vi "SQLite Get Table Names.vi"(8 "error in":errorcluster, 11 "SQLite Connection":refnum<class "Connection.lvclass">) -> (0 "error out":errorcluster, 2 "Table Names":string[](array[string]), 3 "Dup SQLite Connection":refnum<class "Connection.lvclass">)   [LabVIEW 2021, in "EDT SQLite+.lvlib"]
uses:
  EDT SQLite+.lvlib
  <vilib>/drjdpowell/SQLite Library/SQL Connection/Connection.lvclass
  <vilib>/drjdpowell/SQLite Library/SQL Statement/SQL Statement.lvclass/SQL Statement.ctl
  <vilib>/drjdpowell/SQLite Library/SQL Statement/Error Message.vi
  <vilib>/drjdpowell/SQLite Library/SQL Statement/Column String.vi
  <vilib>/drjdpowell/SQLite Library/SQL Statement/SQL Statement.lvclass
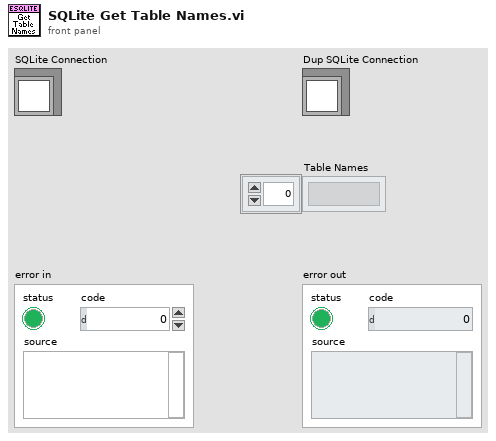
[diagram p1: front panel]
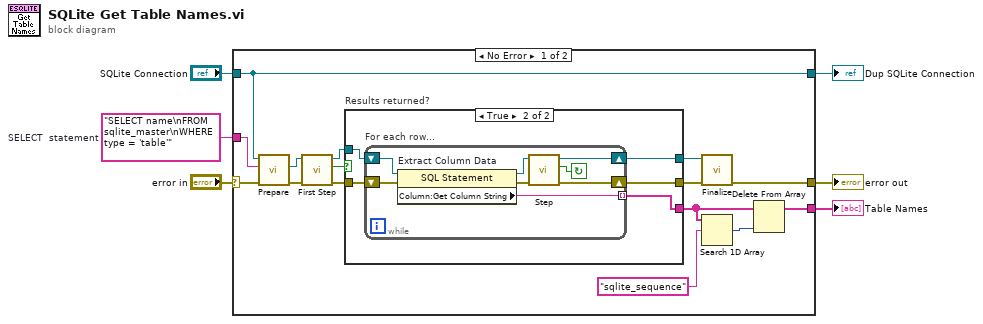
[diagram p0: block diagram]
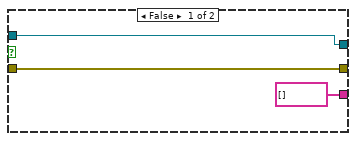
[diagram p2: hidden frame]
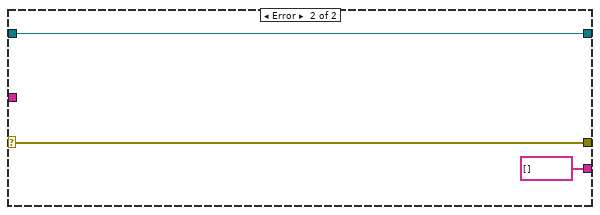
[diagram p3: hidden frame]
diagram:
  w4 = "SELECT name\nFROM sqlite_master\nWHERE type = 'table'"  # SELECT  statement
  n1 = case shown="No Error" "error in" {
    selector: "error in" -> [w21 w40]
    tunnel: [w19 w40] -> w5
    tunnel: "SQLite Connection" -> [w11 w39]
    tunnel: w4 -> [w20 _]
    tunnel: [w11 w39] -> w2
    tunnel: [w7 string[] []] -> w1
    frame No Error {
      n2 = call <vilib>:"Prepare.vi"("error in (no error)"=w21, "SQL"=w20, "SQLite Connection in"=w11) -> ("error out"=w12:errorcluster, "SQL Statement"=w13:refnum<class "SQL Statement.lvclass">)  [unwired: 4 in, 3 out]
      n3 = call <vilib>:"First Step.vi"("error in (no error)"=w12, "SQL Statement in"=w13) -> ("error out"=w15:errorcluster, "Row returned"=w14:bool, "SQL Statement"=w16:refnum<class "SQL Statement.lvclass">)  [unwired: 7 in]
      n4 = case "Results returned?" shown="True" w14 {
        tunnel: [w24 w29] -> w17
        tunnel: [w23 w28] -> w18
        tunnel: w16 -> [w24 w27]
        tunnel: w15 -> [w23 w26]
        tunnel: [string[] [] w25] -> w8
        frame False {
        }
        frame True {
          n5 = while "For each row..." {
            shift-right: [w36] -> w29
            shift-left: w27 -> [w33]
            shift-right: [w34] -> w28
            shift-left: w26 -> [w32]
            tunnel: [w30] -> w25 mode=indexing
            stop <- w31 continue-if-true
            n6 = property on="Extract Column Data" class="SQL Statement"(reference=w33, error in=w32) -> (reference out=w37:refnum<class "SQL Statement.lvclass">, error out=w35:errorcluster, "Column:Get Column String"=w30:string)
            n7 = call <vilib>:"Step.vi"("error in (no error)"=w35, "SQL Statement in"=w37) -> ("error out"=w34:errorcluster, "Row returned"=w31:bool, "SQL Statement"=w36:refnum<class "SQL Statement.lvclass">)  [unwired: 7 in]
          }
        }
      }
      n8 = call <vilib>:"Finalize.vi"("error in (no error)"=w18, "SQL Statement in"=w17) -> ("error out"=w19:errorcluster)  [unwired: 9 in]
      n9 = Search 1D Array(1D array=w8, element="sqlite_sequence") -> (index of element=w9:i32)  [unwired: 1 in]
      n10 = Delete From Array(array=w8, index=w9) -> (array with subset deleted=w7:string[])  [unwired: 1 in, 1 out]
    }
    frame Error {
    }
  }
  "error out" <- w5
  "Dup SQLite Connection" <- w2
  "Table Names" <- w1
